vi "Set Load.vi"(8 "error in (no error)":errorcluster, 10 "load (0)":i32 min=0 max=1000, 11 "VISA resource name":refnum<visa-resource-name>) -> (0 "error out":errorcluster, 3 "VISA resource name out":refnum<visa-resource-name>)   [LabVIEW 2024, in "Revidyne Generator.lvlib"]
doc: "This VI sets the load for the generator. (Accepts values of 0-1000)."
uses:
  Revidyne Generator.lvlib
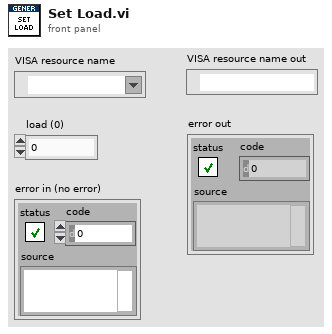
[diagram p1: front panel]
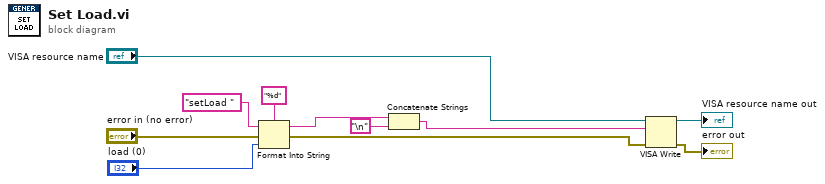
[diagram p0: block diagram]
diagram:
  n1 = Format Into String(format string="%d", initial string="setLoad " ("command"), error in="error in (no error)", "load (0)") -> (resulting string=w3:string, error out=w9:errorcluster)
  n2 = Concatenate Strings(w3, "\n") -> (w2:string)
  n3 = VISA Write(VISA resource name="VISA resource name", write buffer=w2, error in (no error)=w9) -> (VISA resource name out=→"VISA resource name out":refnum<visa-resource-name>, error out=→"error out":errorcluster)  [unwired: 1 out]
